vi "ADC_EASY_Config.vi"(0 "GPIB Address":T4=8, 1 "Trigger mode":T2, 5 "Ch & spans":T3[](array[typedef]) {"low limit (-10V)" format="%.3f"; "high limit (10V)" format="%.3f"}, 7 "buffer size (1000 scans)":u32=1000, 9 "scan rate (1000 scans/sec)":dbl=1000.0 format="%.2f", 11 "error in (no error)":errorcluster) -> (6 "number of channels":i32, 8 "actual scan rate":dbl format="%.2f", 15 "error out":errorcluster)   [LabVIEW 2010]
doc: "This VI configures the hardware and allocates a buffer for a buffered analog input operation for a specified group of channels. \n\nBefore performing any configuration, AI Config checks to see if the input cluster error in indicates that an error has already occurred. If so, then this VI does no configuration, but passes the error information unmodified through error out. In an error condition, taskID is 0.\n\nOtherwise, this VI calls several low-level analog input VIs to set up a task for a buffered analog input acquisition. AI Config calls Analog Input Group Config for the specified device, group, and channels to create a taskID. AI Config then calls Analog Input Hardware Config to record information about the hardware configuration. The input limits input passes to Analog Input Hardware Config, which sets up the lower and upper scaled data limits for each channel; if unspecified, the input limits do not change. This VI configures the number of AMUX boards, the coupling used for each channel (that is, AC, DC, ground, or internal reference), and the input configuration (differential, referenced single-ended, or non-referenced single ended). You can use the low-level Analog Input Hardware Config VI instead if you prefer to specify the input signal range in terms of signal range, polarity, and gain.\n\nAI Config configures the buffer for the acquisition by calling Analog Input Buffer Config. Analog Input Buffer Config allocates memory for the specified number of buffers (the default value is one), where each buffer contains buffer size number of scans.\n\nInput values:\n\n(i32) device: the number of the plug-in data acquisition board. You must specify device. \n\n([string]) channels: specifies the set of analog input channels for a group and task. You cannot assign a channel to more than one group. The default input is channel 0. See the description of the Analog Input Group Config VI for a detailed description of this parameter and the valid syntax for the channel strings.\n\n(i32) buffer size: the number of scans you want each buffer to hold. The default input is 1,000 scans.\n\n(i32) group: the number, from 0 to 15, that you assign to the specified set of channels. The default input and setting for group is 0. If you only have one acquisition for this device, the common case, you can leave this input unwired and use group 0.\n\n([cluster]) input limits: an array of clusters, of which each array element specifies the range limits for the channel(s) in the corresponding element of the channels array. If there are fewer elements in this array than in the channels array, the VI uses the last element for the rest of the channels. The default input is an empty array, which means the input limits do not change from their default settings. Each cluster contains the following parameters: \n\n (sgl) high limit: specifies the maximum scaled data the\n device measures at a particular channel.\n\n (sgl) low limit: specifies the minimum scaled data the\n device measures at a particular channel.\n\n([cluster]) coupling & input config: an array of clusters, of which each array element specifies the coupling and input configuration for the channel(s) in the corresponding element of the channels array. If there are fewer elements in this array than the number of channels, the VI uses the last element for the rest of the channels. The default input is an empty array, which means the parameters do not change from their default settings. Each cluster contains the following parameters: \n\n (u16) coupling: \n 0: Do not change the coupling setting. \n 1: DC. \n 2: AC. \n 3: Ground. \n 4: Internal reference. \n\n (u16) input config: \n 0: Do not change the input config setting. \n 1: Differential. \n 2: Referenced single-ended. \n 3: Nonreferenced single-ended. \n\n(sgl) Interchannel delay in seconds is the interval of time between two channels being sampled in your channel list.\n\n\n(i32) number of buffers: the number of buffers the VI allocates. The default input is 1 and you need to change it only for multi-buffered acquisition.\n\n(i32) number of AMUX: the number of AMUX-64T boards attached, either 0, 1, 2, or 4.\n\n(cluster) error in: a cluster describing any error conditions prior to this VI's execution. The default input of this cluster is no error. AI Config is often the first subVI in your diagram, and you may not need to wire this input. If an error has already occurred, this VI does not do the input configuration, it just passes the values of taskID in and error in to taskID out and error out. The error in cluster contains the following parameters: \n\n (bool) status: TRUE if an error has occurred.\n If status is TRUE, this VI does not do the\n input configuration.\n\n (i32) code: the error code associated with an error.\n A value of 0 means no error, a negative value is an error,\n and a positive value is a warning.\n\n (string) source: an indication of where an \n error occurred, usually the name of the VI.\n\nOutput Values:\n\n(u32) taskID: uniquely identifies the device, group, and I/O operation. Use this value as taskID in to refer to this group's operation in subsequent VIs.\n\n(i32) number of channels: the total number of channels that belong to the group, including any AMUX or SCXI channels.\n\n(cluster) error out: a cluster containing error information. If error in indicated an error, error out contains the same error information. Otherwise, it describes the error status of this VI. Use the General Error Handler utility VI to check the error at the end of your diagram. The error out cluster contains the following parameters: \n\n (bool) status: TRUE if an error has occurred.\n\n (i32) code: the error code associated with an error.\n A value of 0 means no error, a negative value is an error,\n and a positive value is a warning.\n\n (string) source: an indication of where an \n error occurred, usually the name of the VI."
uses:
  ADC_GPIB_address.ctl
  Controls/Ch_and_Spans.ctl
  Controls/Trigger_Mode.ctl
panel:
  in  "Trigger override":bool
  in  "Trigger Spec":T1={"level %(1.00)"=50.0, "slope"=enum."Rising", "Source"=enum."External TTL", "pretrigger scans (0)"=0} {"level %(1.00)" min=-100 max=100 step=1}
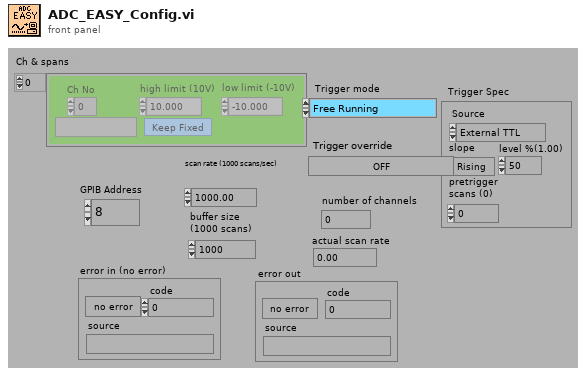
[diagram p1: front panel]
types:
  T1 = cluster{"level %(1.00)":sgl, "slope":enum16{"Rising", "Falling"}, "Source":enum16{"Free running..", "GPIB GET", "External TTL", "First Channel", "One shot on TALK", "On shot on GET", "One shot TTL"}, "pretrigger scans (0)":u32}
  T2 = typedef "Trigger_Mode.ctl" = enum16{"Free Running", "Start on Trigger", "Trigger Every Block", "Trigger Every Sample"}
  T3 = typedef "Ch_and_Spans.ctl" = cluster{"high limit (10V)":sgl, "low limit (-10V)":sgl, "Ch No":i16, "Var name":string, "Use Latest Calib":bool}
  T4 = typedef "ADC_GPIB_address.ctl" = u8
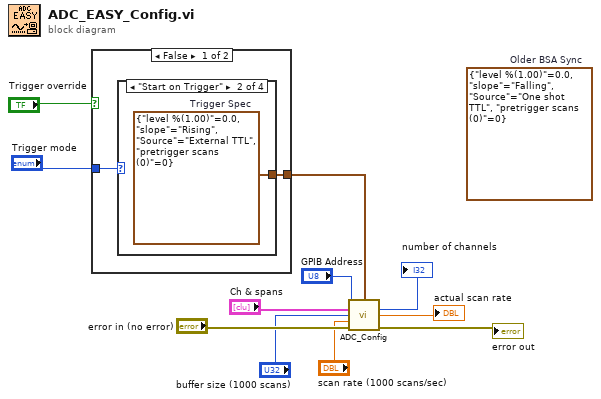
[diagram p0: block diagram]
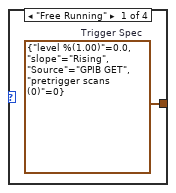
[diagram p2: hidden frame]
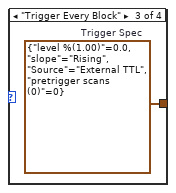
[diagram p3: hidden frame]
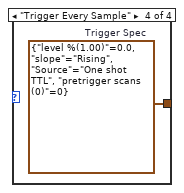
[diagram p4: hidden frame]
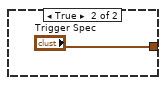
[diagram p5: hidden frame]
diagram:
  (unwired) T1 {"level %(1.00)"=0.0, "slope"=enum."Falling", "Source"=enum."One shot TTL", "pretrigger scans (0)"=0}  # Older BSA Sync
  n1 = case shown="False" "Trigger override" {
    tunnel: [w13 "Trigger Spec"] -> w5
    tunnel: "Trigger mode" -> [w12 _]
    frame False {
      n2 = case shown="\"Start on Trigger\"" w12 {
        tunnel: [w14 w15 w16 w17] -> w13
        frame "Free Running" {
          w14 = T1 {"level %(1.00)"=0.0, "slope"=enum."Rising", "Source"=enum."GPIB GET", "pretrigger scans (0)"=0}  # Trigger Spec
        }
        frame "Start on Trigger" {
          w15 = T1 {"level %(1.00)"=0.0, "slope"=enum."Rising", "Source"=enum."External TTL", "pretrigger scans (0)"=0}  # Trigger Spec
        }
        frame "Trigger Every Block" {
          w16 = T1 {"level %(1.00)"=0.0, "slope"=enum."Rising", "Source"=enum."External TTL", "pretrigger scans (0)"=0}  # Trigger Spec
        }
        frame "Trigger Every Sample" {
          w17 = T1 {"level %(1.00)"=0.0, "slope"=enum."Rising", "Source"=enum."One shot TTL", "pretrigger scans (0)"=0}  # Trigger Spec
        }
      }
    }
    frame True {
    }
  }
  n3 = call "ADC_Config.vi"("GPIB Address"="GPIB Address", "Trigger Spec"=w5, "Ch & spans"="Ch & spans", "buffer size (1000 scans)"="buffer size (1000 scans)", "scan rate (1000 scans/sec)"="scan rate (1000 scans/sec)", "error in (no error)"="error in (no error)") -> ("number of channels"=→"number of channels":i32, "actual scan rate"=→"actual scan rate":dbl, "error out"=→"error out":errorcluster)  [unwired: 7 out]
